vi "sha256_scram_client_first.vi"(10 "password":string, 11 "user":string) -> (3 "client_first_message":string)   [LabVIEW 2019, in "hashlib.lvlib"]
doc: "Calculates the <b>SCRAM-SHA-256 FIRST CLIENT MESSAGE</b> to send to the server for web authentication based on the <b>user</b> and <b>password</b>. The password is salted with random bytes prior to formatting the first message.\n\nRFC 5802\n\nCreated by: Ryan Pacini"
uses:
  hashlib.lvlib
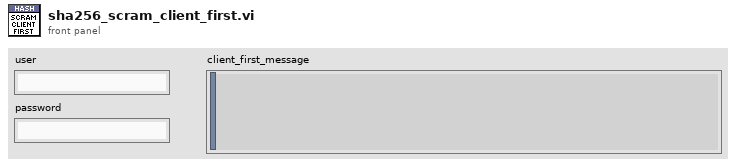
[diagram p1: front panel]
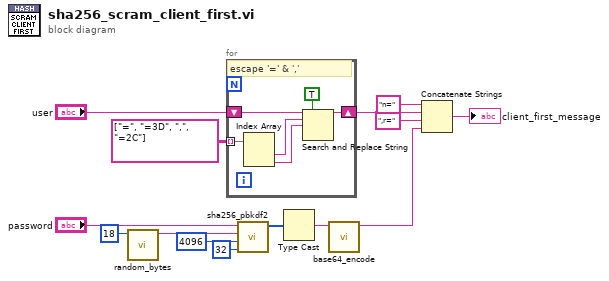
[diagram p0: block diagram]
diagram:
  n1 = call "random_bytes.vi"("length (18bytes)"=18 ("length")) -> ("random bytes"=w7:string)  [unwired: 10 in]
  n2 = for {
    shift-right: [w19] -> w4
    shift-left: "user" -> [w20]
    tunnel: string[][] [["=", "=3D"], [",", "=2C"]] -> [w17] mode=indexing
    # "escape '=' & ','"
    n3 = Index Array(array=w17) -> (element #1=w16:string, element #2=w15:string)  [unwired: 2 in]
    n4 = Search and Replace String(replace all?=TRUE ("replace all? (F)"), input string=w20, search string=w16, replace string=w15) -> (result string=w19:string)  [unwired: 4 in, 3 out]
  }
  n5 = call "sha256_pbkdf2.vi"("dkLen (32octets=sha256)"=32, "iterations"=4096, "salt"=w7, "password"="password") -> ("sha-256"=w5:u32[])  [unwired: 7 in]
  n6 = Type Cast(x=w5) -> (*(type *) &x=w11:string)  [unwired: 1 in]
  n7 = call "base64_encode.vi"("string"=w11) -> ("base64"=w3:string)  [unwired: 10 in]
  n8 = Concatenate Strings("n=" ("string"), w4, ",r=" ("string"), w3) -> (→"client_first_message":string)
